vi "get_fav_place.vi"() -> (4 "place":T2, 6 "Back out":T1, 8 "path":path)   [LabVIEW 2023]
doc: "Get the place from user"
uses:
  custom_elements/fav_places.ctl
  custom_elements/back_button.ctl
panel:
  in  "Back":T1
  in  "home":bool caption="Home"
  in  "beach":bool caption="Beach"
  in  "mountain":bool caption="Mountain"
  in  "Forest":bool
  # "Select you favourite Place"
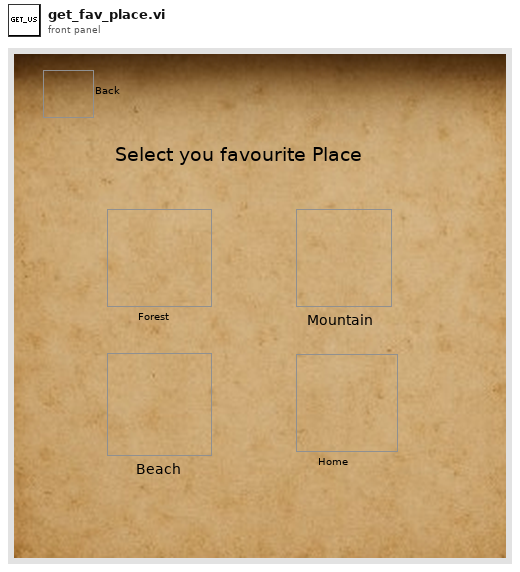
[diagram p1: front panel]
types:
  T1 = typedef "back_button.ctl" = bool
  T2 = typedef "fav_places.ctl" = enum16{"Forest", "Mountain", "Beach", "Home"}
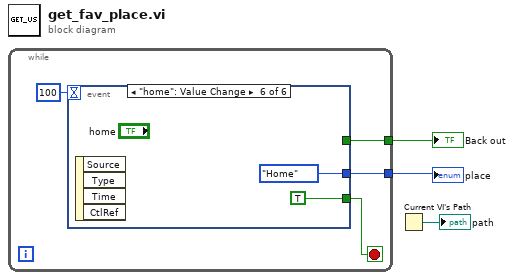
[diagram p0: block diagram]
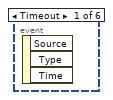
[diagram p2: hidden frame]
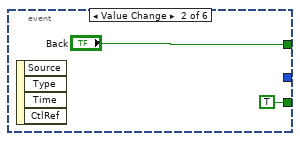
[diagram p3: hidden frame]
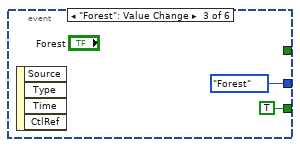
[diagram p4: hidden frame]
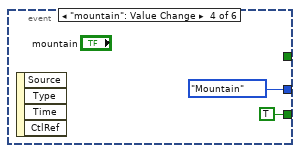
[diagram p5: hidden frame]
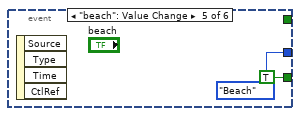
[diagram p6: hidden frame]
diagram:
  n1 = while {
    tunnel: [w5] -> w2
    tunnel: [w4] -> w1
    stop <- w6 stop-if-true
    n2 = event shown="[5] \"home\": Value Change" {
      selector: _ -> [_ _ _ _ _ _]
      dyn-events: _ -> [_ _ _ _ _ _]
      timeout: 100 -> [_ _ _ _ _ _]
      tunnel: [_ TRUE TRUE TRUE TRUE TRUE] -> w6
      tunnel: [_ _ enum16{"Forest", "Mountain", "Beach", "Home"}."Forest" ("Enum") enum16{"Forest", "Mountain", "Beach", "Home"}."Mountain" ("Enum") enum16{"Forest", "Mountain", "Beach", "Home"}."Beach" ("Enum") enum16{"Forest", "Mountain", "Beach", "Home"}."Home" ("Enum")] -> w5
      tunnel: [_ "Back" _ _ _ _] -> w4
      event Timeout {
        n3 = event-data() -> ()  [unwired: 1 in, 3 out]
      }
      event Value Change {
        n4 = event-data() -> ()  [unwired: 1 in, 4 out]
      }
      event "Forest": Value Change {
        n5 = event-data() -> ()  [unwired: 1 in, 4 out]
      }
      event "mountain": Value Change {
        n6 = event-data() -> ()  [unwired: 1 in, 4 out]
      }
      event "beach": Value Change {
        n7 = event-data() -> ()  [unwired: 1 in, 4 out]
      }
      event "home": Value Change {
        n8 = event-data() -> ()  [unwired: 1 in, 4 out]
      }
    }
  }
  "place" <- w2
  "Back out" <- w1
  n9 = Current VI's Path() -> (path=→"path":path)
